vi "test (Example).vi"(8 "error in (no error)":errorcluster, 11 "Parentheses (Valid).lvclass":refnum<class "Parentheses (Valid).lvclass">) -> (0 "error out":errorcluster, 3 "Parentheses (Valid).lvclass":refnum<class "Parentheses (Valid).lvclass">)   [LabVIEW 2013, in "Parentheses (Valid).lvclass"]
uses:
  Parentheses (Valid).lvclass
  Classes/TestCase/TestCase.lvclass
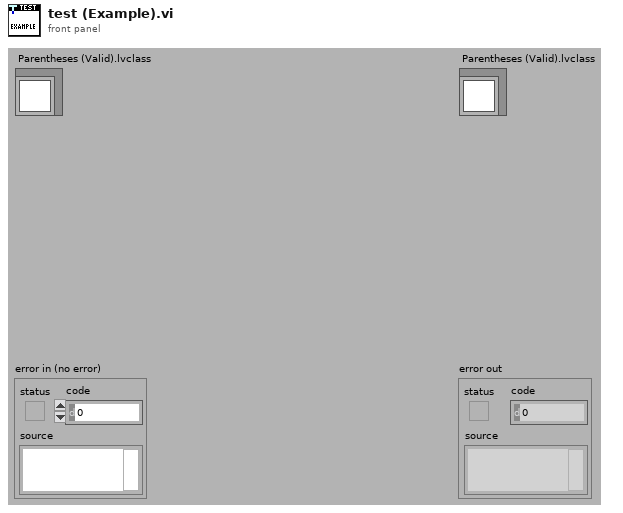
[diagram p1: front panel]
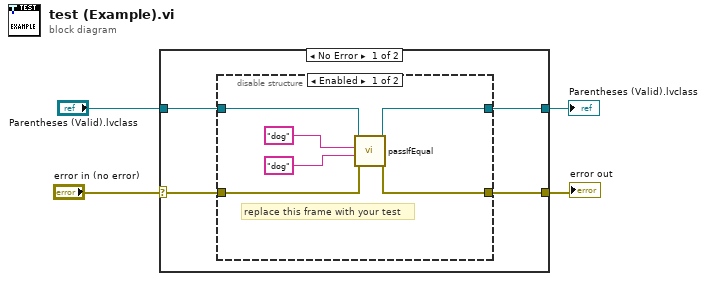
[diagram p0: block diagram]
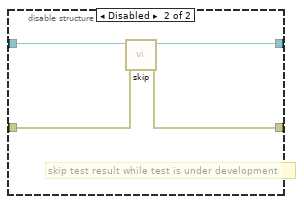
[diagram p2: hidden frame]
diagram:
  n1 = case shown="No Error" "error in (no error)" {
    selector: "error in (no error)" -> [w6 w20]
    tunnel: [w5 w20] -> w3
    tunnel: [w7 w19] -> w1
    tunnel: "Parentheses (Valid).lvclass" -> [w8 w19]
    frame No Error {
      n2 = disable-structure shown="Enabled" {
        disable-tunnel: w8 -> [w12 w18]
        disable-tunnel: [w11 w15] -> w7
        disable-tunnel: w6 -> [w10 w17]
        disable-tunnel: [w9 w16] -> w5
        frame Enabled {
          # "replace this frame with your test"
          n3 = call-dynamic "passIfEqual.vi"("error in (no error)"=w10, "y"="dog", "x"="dog", "TestCase in"=w12) -> ("error out"=w9:errorcluster, "TestCase out"=w11:refnum<class "Parentheses (Valid).lvclass">)  [unwired: 6 in]
        }
        frame Disabled {
          # "skip test result while test is under development"
          n4 = call "skip.vi"("error in (no error)"=w17, "TestCase in"=w18) -> ("error out"=w16:errorcluster, "TestCase out"=w15:refnum<class "Parentheses (Valid).lvclass">)  [unwired: 8 in]
        }
      }
    }
    frame Error {
    }
  }
  "error out" <- w3
  "Parentheses (Valid).lvclass" <- w1
